vi "Middle Rail.vi"(11 "Full System Configuration":T1={"Rack"=enum."15U; 1-Phase; 16A; 100-240V", "Middle Rail"=enum."None", "Ballast"={"Main"=0, "Small"=0, "Side"=0}, "Front Panel I/O"={"EMO Button"=FALSE, "USB 3.0"=FALSE, "Display"=FALSE, "1st USB 2.0"=FALSE, "2nd USB 2.0"=FALSE, "Ethernet 3"=FALSE, "EMO Extension (3rd Party)"=FALSE, "EMO Extension (Rack In & Out)"=FALSE, "Aux Dual C13 QAC Outlets"=FALSE, "Residual-current Circuit Breaker"=FALSE, "Serial"=FALSE, "GPIB"=FALSE}, "Rear Panel I/O"={"Rear Panel I/O Configuration"=enum."Blank Panel", "EMO Button"=FALSE, "Power, Status & Banana Ground"=FALSE, "Ethernet 2"=FALSE, "Display"=FALSE, "USB 3.0"=FALSE, "DIO"=FALSE, "GPIB"=FALSE, "Aux Dual C13 QAC Outlets"=FALSE, "Residual-current Circuit Breaker"=FALSE, "Serial"=FALSE, "SMA"=FALSE}, "Miscellaneous Options"={"Eyebolts"=FALSE, "Tower Light"=FALSE, "Top/Side Monitor Mount Kit"=FALSE, "24\" Monitor"=FALSE, "Keyboard & Mouse"=FALSE, "Secondary Ethernet Switch"=FALSE, "Extra USB Hub"=FALSE, "USB-6509"=FALSE, "Front Door"=enum."38U (Solid) IG", "Primary Ethernet Switch"=enum."Item 0", "Use Posture"=enum."Item 0"}, "Accessories"={"Screw Type"=enum."10-32", "Cage Nuts & Screws"=0.0, "Filler Panel Color"=enum."Interface Gray", "1U"=0.0, "2U"=0.0, "3U"=0.0}} {"Ballast"."Side" max=5 step=1; "Ballast"."Small" max=5 step=1; "Ballast"."Main" max=5 step=1}) -> (2 "cluster":T13)   [LabVIEW 2023]
uses:
  Option Type Defs/Parts List.ctl
  Option Type Defs/Full System Configuration.ctl
  Option Type Defs/Rack.ctl
  Option Type Defs/Middle Rail.ctl
  Option Type Defs/Ballast.ctl
  Option Type Defs/Front Panel IO.ctl
  Option Type Defs/Rear Panel IO.ctl
  Option Type Defs/Rear Panel IO Configuration.ctl
  Option Type Defs/Miscellaneous Options.ctl
  Option Type Defs/Front Door.ctl
  <userlib>/_OpenG.lib/lvdata/lvdata.llb/openg_variant.lvlib
  Option Type Defs/Screw Types.ctl
  Option Type Defs/Filler Panel Color.ctl
  Option Type Defs/Accessories.ctl
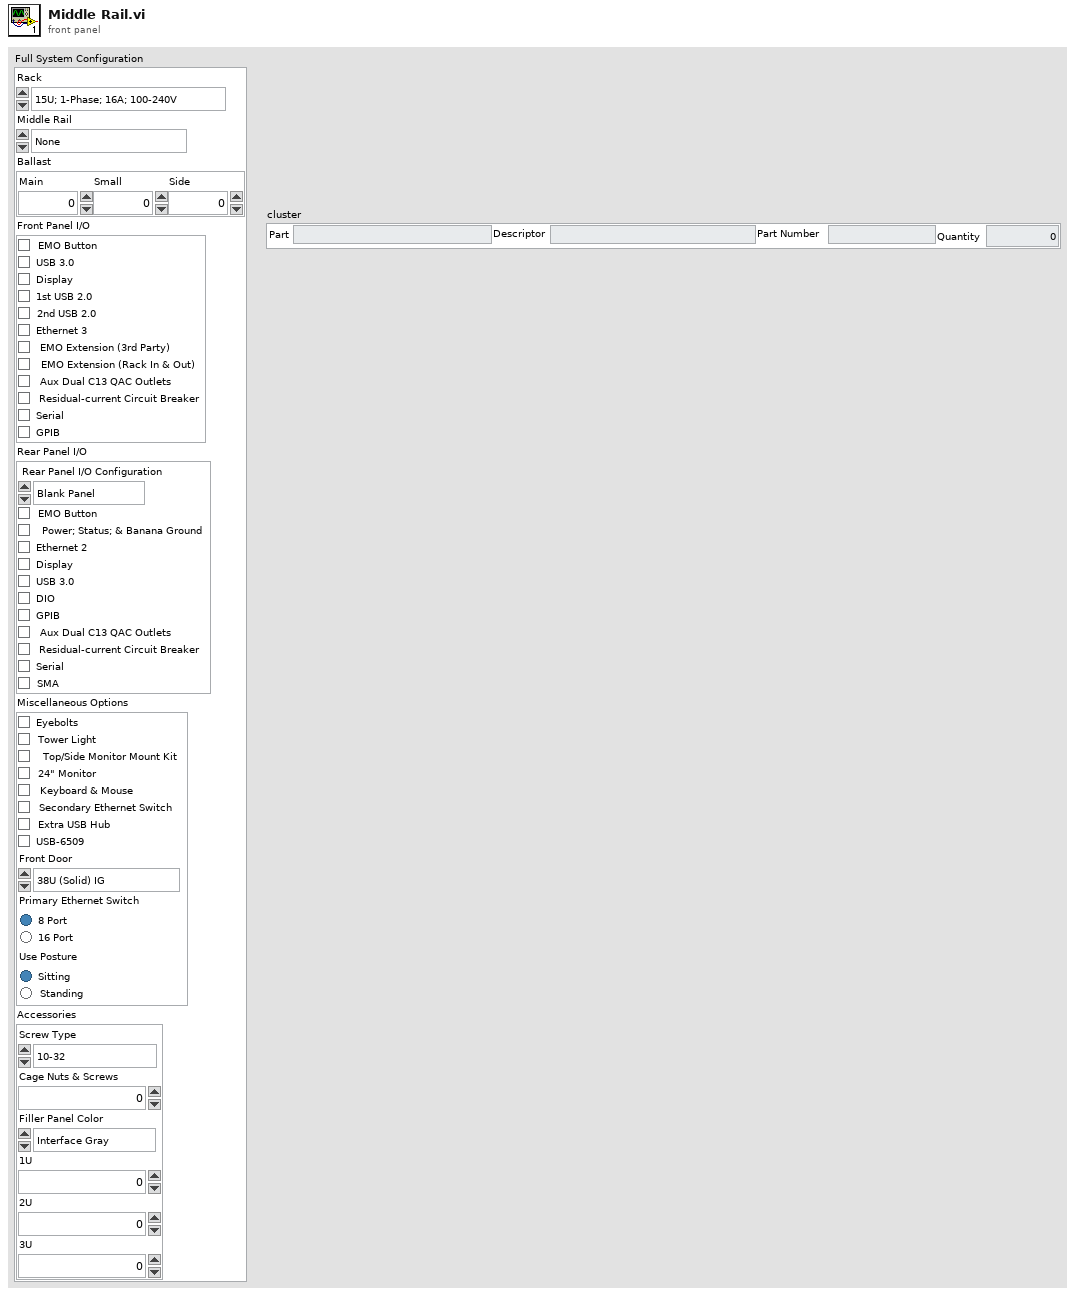
[diagram p1: front panel]
types:
  T1 = typedef "Full System Configuration.ctl" = cluster{"Rack":T2, "Middle Rail":T3, "Ballast":T4, "Front Panel I/O":T5, "Rear Panel I/O":T6, "Miscellaneous Options":T8, "Accessories":T10}
  T2 = typedef "Rack.ctl" = enum16{"15U; 1-Phase; 16A; 100-240V", "15U; 1-Phase; 24A; 100-240V", "38U; 3-Phase Delta; 50A; 200-240V", "38U; 1-Phase; 24A; 100-120V", "38U; 3-Phase Wye; 50A; 200-240V", "38U; 3-Phase Delta; 50A; 380-480V", "38U; 3-Phase Delta; 32A; 200-240V", "38U; 3-Phase Wye; 16A; 100-240V", "44U; 1-Phase; 24A; 100-240V", "44U; 3-Phase Delta; 32A; 200-240V"}
  T3 = typedef "Middle Rail.ctl" = enum16{"None", "Flip Side Rear; D=168.83mm", "Parallel Rear; D=145mm", "Flip Side Front; D=145mm", "Parallel Front; D=145mm"}
  T4 = typedef "Ballast.ctl" = cluster{"Main":u16, "Small":u16, "Side":u16}
  T5 = typedef "Front Panel IO.ctl" = cluster{"EMO Button":bool, "USB 3.0":bool, "Display":bool, "1st USB 2.0":bool, "2nd USB 2.0":bool, "Ethernet 3":bool, "EMO Extension (3rd Party)":bool, "EMO Extension (Rack In & Out)":bool, "Aux Dual C13 QAC Outlets":bool, "Residual-current Circuit Breaker":bool, "Serial":bool, "GPIB":bool}
  T6 = typedef "Rear Panel IO.ctl" = cluster{"Rear Panel I/O Configuration":T7, "EMO Button":bool, "Power, Status & Banana Ground":bool, "Ethernet 2":bool, "Display":bool, "USB 3.0":bool, "DIO":bool, "GPIB":bool, "Aux Dual C13 QAC Outlets":bool, "Residual-current Circuit Breaker":bool, "Serial":bool, "SMA":bool}
  T7 = typedef "Rear Panel IO Configuration.ctl" = enum16{"Blank Panel", "Fully Populated Panel", "Custom Panel"}
  T8 = typedef "Miscellaneous Options.ctl" = cluster{"Eyebolts":bool, "Tower Light":bool, "Top/Side Monitor Mount Kit":bool, "24\" Monitor":bool, "Keyboard & Mouse":bool, "Secondary Ethernet Switch":bool, "Extra USB Hub":bool, "USB-6509":bool, "Front Door":T9, "Primary Ethernet Switch":enum32{"Item 0", "Item 1"}, "Use Posture":enum32{"Item 0", "Item 1"}}
  T9 = typedef "Front Door.ctl" = enum16{"None", "38U (Solid) IG", "38U (Solid) EG", "38U: Top 14U (Solid) IG", "38U (Clear) IG", "44U (Solid) IG", "44U (Solid) EG"}
  T10 = typedef "Accessories.ctl" = cluster{"Screw Type":T11, "Cage Nuts & Screws":dbl, "Filler Panel Color":T12, "1U":dbl, "2U":dbl, "3U":dbl}
  T11 = typedef "Screw Types.ctl" = enum16{"None", "M6 (Most Common)", "10-32", "12-24"}
  T12 = typedef "Filler Panel Color.ctl" = enum16{"None", "Interface Gray", "Environmental Gray"}
  T13 = typedef "Parts List.ctl" = cluster{"Part":string, "Descriptor":string, "Part Number":string, "Quantity":dbl}
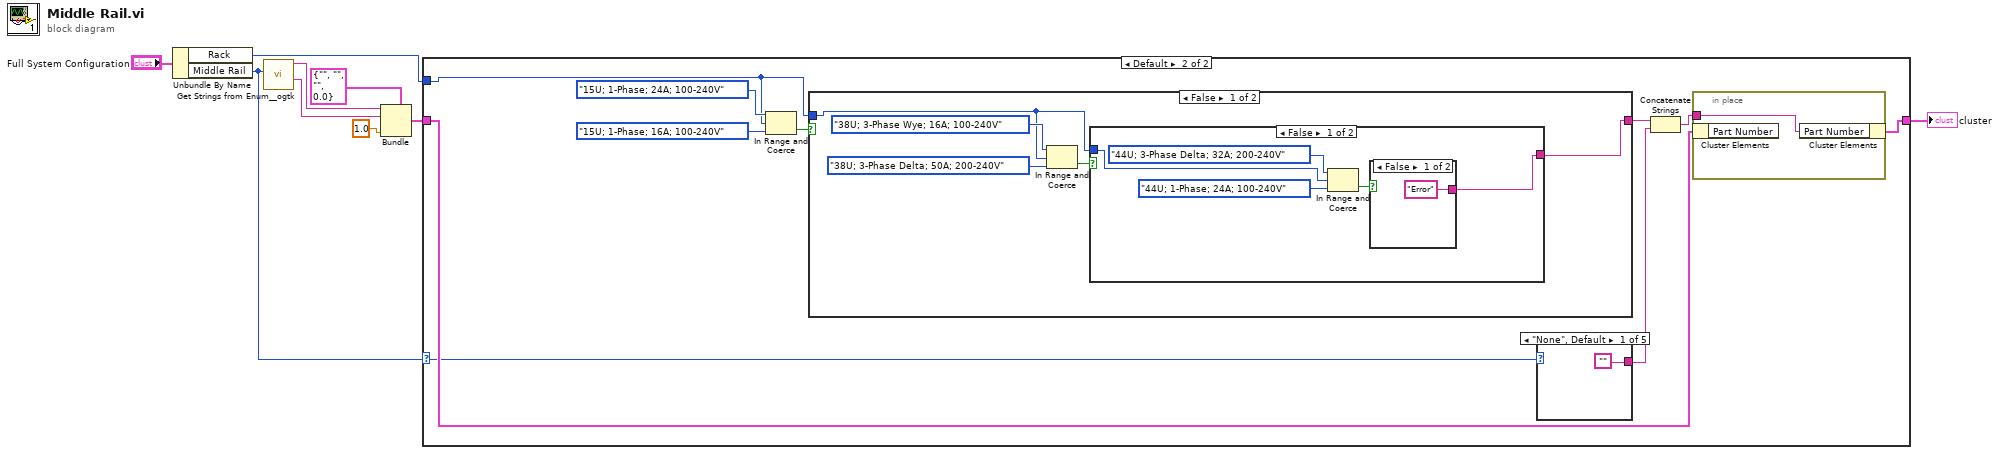
[diagram p0: block diagram]
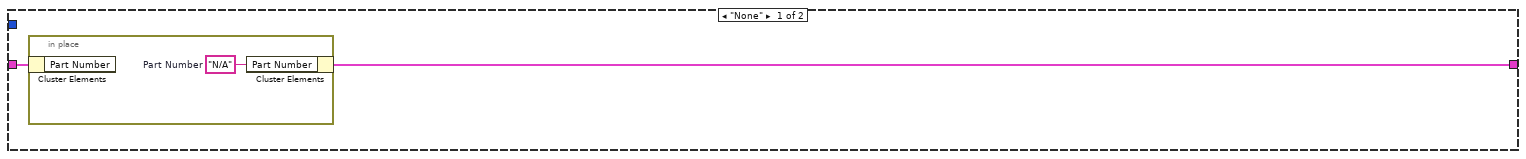
[diagram p2: hidden frame]
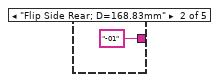
[diagram p3: hidden frame]
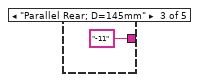
[diagram p4: hidden frame]
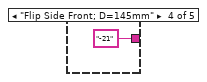
[diagram p5: hidden frame]
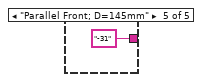
[diagram p6: hidden frame]
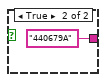
[diagram p7: hidden frame]
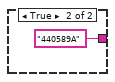
[diagram p8: hidden frame]
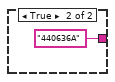
[diagram p9: hidden frame]
diagram:
  n1 = Unbundle By Name("Full System Configuration") -> ("Rack"=w8:T2, "Middle Rail"=w7:T3)
  n2 = call <userlib>:"Get Strings from Enum__ogtk.vi"("Enum"=w7) -> ("String Value"=w5:string, "Enum Name"=w4:string)  [unwired: 7 in, 2 out]
  n3 = Bundle(cluster=T13 {"Part"="", "Descriptor"="", "Part Number"="", "Quantity"=0.0}, "Part"=w4, "Descriptor"=w5, "Quantity"=1.0) -> (w6:T13)  [unwired: 1 in]
  n4 = case shown="Default" w7 {
    selector: w7 -> [_ w17]
    tunnel: w6 -> [w11 w22]
    tunnel: w8 -> [_ w13]
    tunnel: [w10 w19] -> w9
    frame "None" {
      n5 = in-place {
        w12 = "N/A"  # Part Number
        n6 = in-place-cluster #1(w11) -> ()  [unwired: 1 out]
        n7 = in-place-cluster #1("Part Number"=w12) -> (w10:T13)
      }
    }
    frame Default {
      n8 = In Range and Coerce(upper limit=Rack."15U; 1-Phase; 24A; 100-240V" ("Rack"), x=w13, lower limit=Rack."15U; 1-Phase; 16A; 100-240V" ("Rack")) -> (In Range?=w14:bool)  [unwired: 1 out]
      n9 = case shown="False" w14 {
        tunnel: [w32 "440636A"] -> w21
        tunnel: w13 -> [w28 _]
        frame False {
          n10 = In Range and Coerce(upper limit=Rack."38U; 3-Phase Wye; 16A; 100-240V" ("Rack"), x=w28, lower limit=Rack."38U; 3-Phase Delta; 50A; 200-240V" ("Rack")) -> (In Range?=w29:bool)  [unwired: 1 out]
          n11 = case shown="False" w29 {
            tunnel: [w33 "440589A"] -> w32
            tunnel: w28 -> [w35 _]
            frame False {
              n12 = In Range and Coerce(upper limit=Rack."44U; 3-Phase Delta; 32A; 200-240V" ("Rack"), x=w35, lower limit=Rack."44U; 1-Phase; 24A; 100-240V" ("Rack")) -> (In Range?=w34:bool)  [unwired: 1 out]
              n13 = case shown="False" w34 {
                tunnel: ["Error" "440679A"] -> w33
                frame False {
                }
                frame True {
                }
              }
            }
            frame True {
            }
          }
        }
        frame True {
        }
      }
      n14 = case shown="\"None\", Default" w17 {
        tunnel: ["" "-01" "-11" "-21" "-31"] -> w18
        frame "None", Default {
        }
        frame "Flip Side Rear; D=168.83mm" {
        }
        frame "Parallel Rear; D=145mm" {
        }
        frame "Flip Side Front; D=145mm" {
        }
        frame "Parallel Front; D=145mm" {
        }
      }
      n15 = Concatenate Strings(w21, w18) -> (w20:string)
      n16 = in-place {
        in-place-border: w20 -> [w42]
        n17 = in-place-cluster #2(w22) -> ()  [unwired: 1 out]
        n18 = in-place-cluster #2("Part Number"=w42) -> (w19:T13)
      }
    }
  }
  "cluster" <- w9
